vi "Express VI - Amplitude and Level Measurements.vi"() -> ()   [LabVIEW 2023]
doc: "This example shows how to take some amplitude measurements on a simulated signal. The measurements are Mean (DC) and RMS.\n\nThis example uses the following Express VIs: Simulate Signal and Amplitude and Level Measurements"
uses:
  Instance           2 36Saved   Basic Amplitude Measurements .vi
  Instance           3 36Saved   Basic Amplitude Measurements .vi
panel:
  in  "Frequency":dbl(slide)=40.39408866995074 scale=0.0..100.0
  out "RMS":dbl format="%.2f"
  out "Mean":dbl format="%.2f"
  in  "Amplitude":dbl(slide)=10.0 scale=0.0..10.0
  out "Input":dynamicdata(graph)
  in  "Stop":bool
  # "Overview: Demonstrates how to take some amplitude measurements on a simulated signal.\nRequirements: LabVIEW Full Development System\nInstructions:\n1. Run the VI.\n2. Change the frequency and the amplitude with the sliders.\n3. Click Stop to stop the VI."
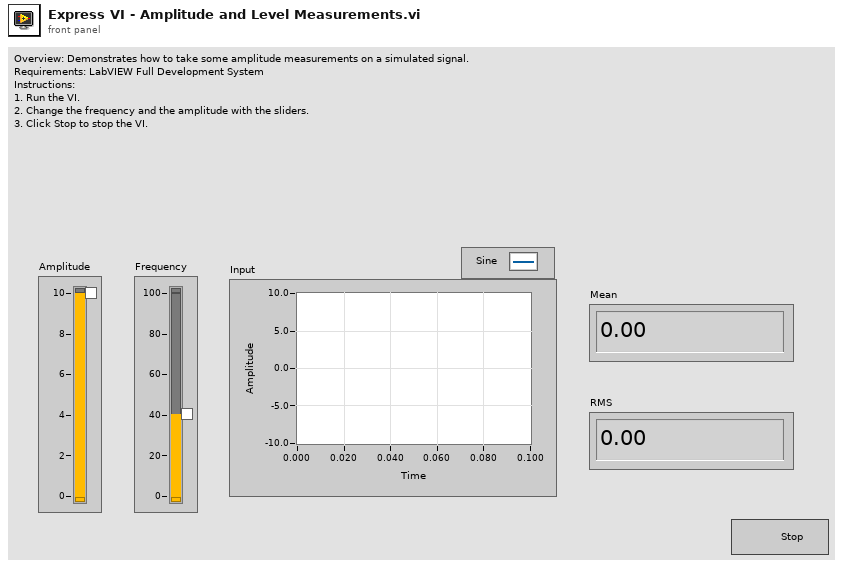
[diagram p1: front panel]
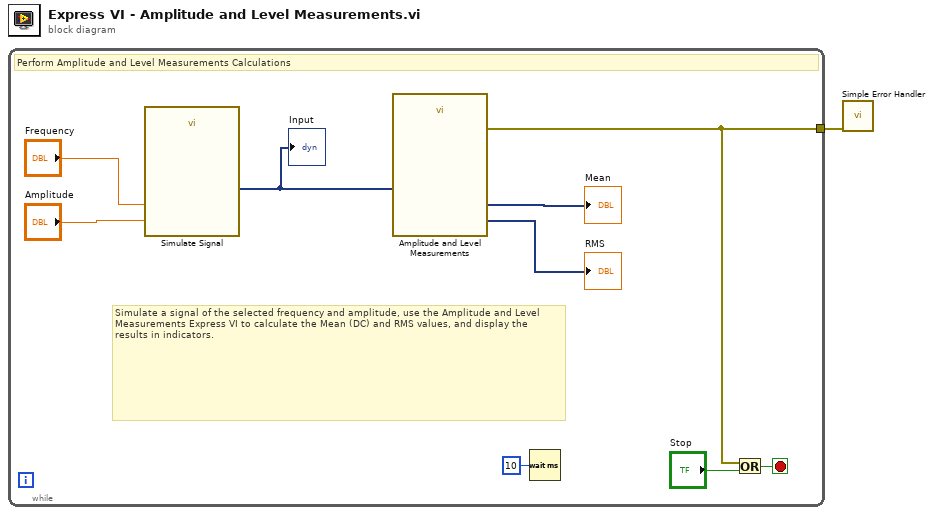
[diagram p0: block diagram]
diagram:
  n1 = while {
    tunnel: [w2] -> w1
    stop <- w4 stop-if-true
    # "Simulate a signal of the selected frequency and amplitude, use the Amplitude and Level Measurements Express VI to calculate the Mean (DC) and RMS values, and display the results in indicators."
    # "Perform Amplitude and Level Measurements Calculations"
    n2 = call "Simulate Signal"("Frequency"="Frequency", "Amplitude"="Amplitude") -> ("Sine"=w8:dynamicdata)  [unwired: 4 in, 9 out]
    "Input" <- w8
    n3 = call "Amplitude and Level Measurements"("Signals"=w8) -> ("Mean (DC)"=→"Mean":dynamicdata, "RMS"=→"RMS":dynamicdata, "error out"=w2:errorcluster)  [unwired: 2 in, 10 out]
    n4 = Wait (ms)(milliseconds to wait=u32 10) -> ()  [unwired: 1 out]
    n5 = Or(x=w2, y="Stop") -> (x .or. y?=w4:bool)
  }
  n6 = call <vilib>:"Simple Error Handler.vi"("error in (no error)"=w1) -> ()  [unwired: 4 in, 5 out]
